vi "引用測試5.vi"() -> ()   [LabVIEW 2015]
uses:
  <vilib>/vision/Measure.llb/Edge Options.ctl
  <vilib>/vision/Measure.llb/Edge Polarity.ctl
  <vilib>/userdefined/High Color/IMAQdx.ctl
  <vilib>/vision/driver/NI_Vision_Acquisition_Software.lvlib
  <vilib>/vision/NI_Vision_Development_Module.lvlib
panel:
  out "Line Profile":T1(graph)
  out "Location (Pixel)":cluster{"X":sgl, "Y":sgl}
  in  "線":enum16{"Start to End", "End to Start"}(ring)
  in  "Session In":T2="cam0"
  out "output cluster":cluster{"Data name":string, "Data":variant}
  in  "Numeric":i32
  in  "ROI":T3=enum."Set Data"
  in  "動作":bool
  in  "重新開圖":bool
  out "Line Data":cluster{"X":sgl, "Y":sgl, "T":sgl}
  in  "開圖":bool
  in  "ShowData":bool
  in  "DieArea":i32=100 min=10
  in  "動作":enum16{"什麼也不做", "抓邊", "看灰階", "分析光源均勻度"}(ring)
  out "Mean":sgl format="%#.2f"
  out "Histogram":T4(graph)
  in  "取像":bool
  in  "Edge Options":T5={"Edge Polarity"=0, "Kernel Size"=3, "Width"=3, "Minimum Edge Strength"=10.0, "Interpolation Type"=enum."Bilinear Fixed", "Data Processing Method"=enum."Average"} {"Edge Polarity" items=["All Edges", "Rising Edges", "Falling Edges"]; "Minimum Edge Strength" format="%.2f"; "Width" step=2; "Kernel Size" step=2}
  out "error out":errorcluster
  out "Ellipse":T7 {"Minor Axis"."Point 2"."Y" format="%.2f"; "Minor Axis"."Point 2"."X" format="%.2f"; "Minor Axis"."Point 1"."Y" format="%.2f"; "Minor Axis"."Point 1"."X" format="%.2f"; "Major Axis"."Point 2"."Y" format="%.2f"; "Major Axis"."Point 2"."X" format="%.2f"; "Major Axis"."Point 1"."Y" format="%.2f"; "Major Axis"."Point 1"."X" format="%.2f"; "Center"."Y" format="%.2f"; "Center"."X" format="%.2f"}
  in  "圓":enum16{"Inner to Outer", "Outer to Inner"}(ring)
  out "Gradient Information":dbl[][](graph)
  in  "邊":T8(ring)
  in  "Process":T9(ring)
  in  "Gap":i32=10 min=1 max=300
  in  "stop":bool
  out "Image":T10(plugin-control)
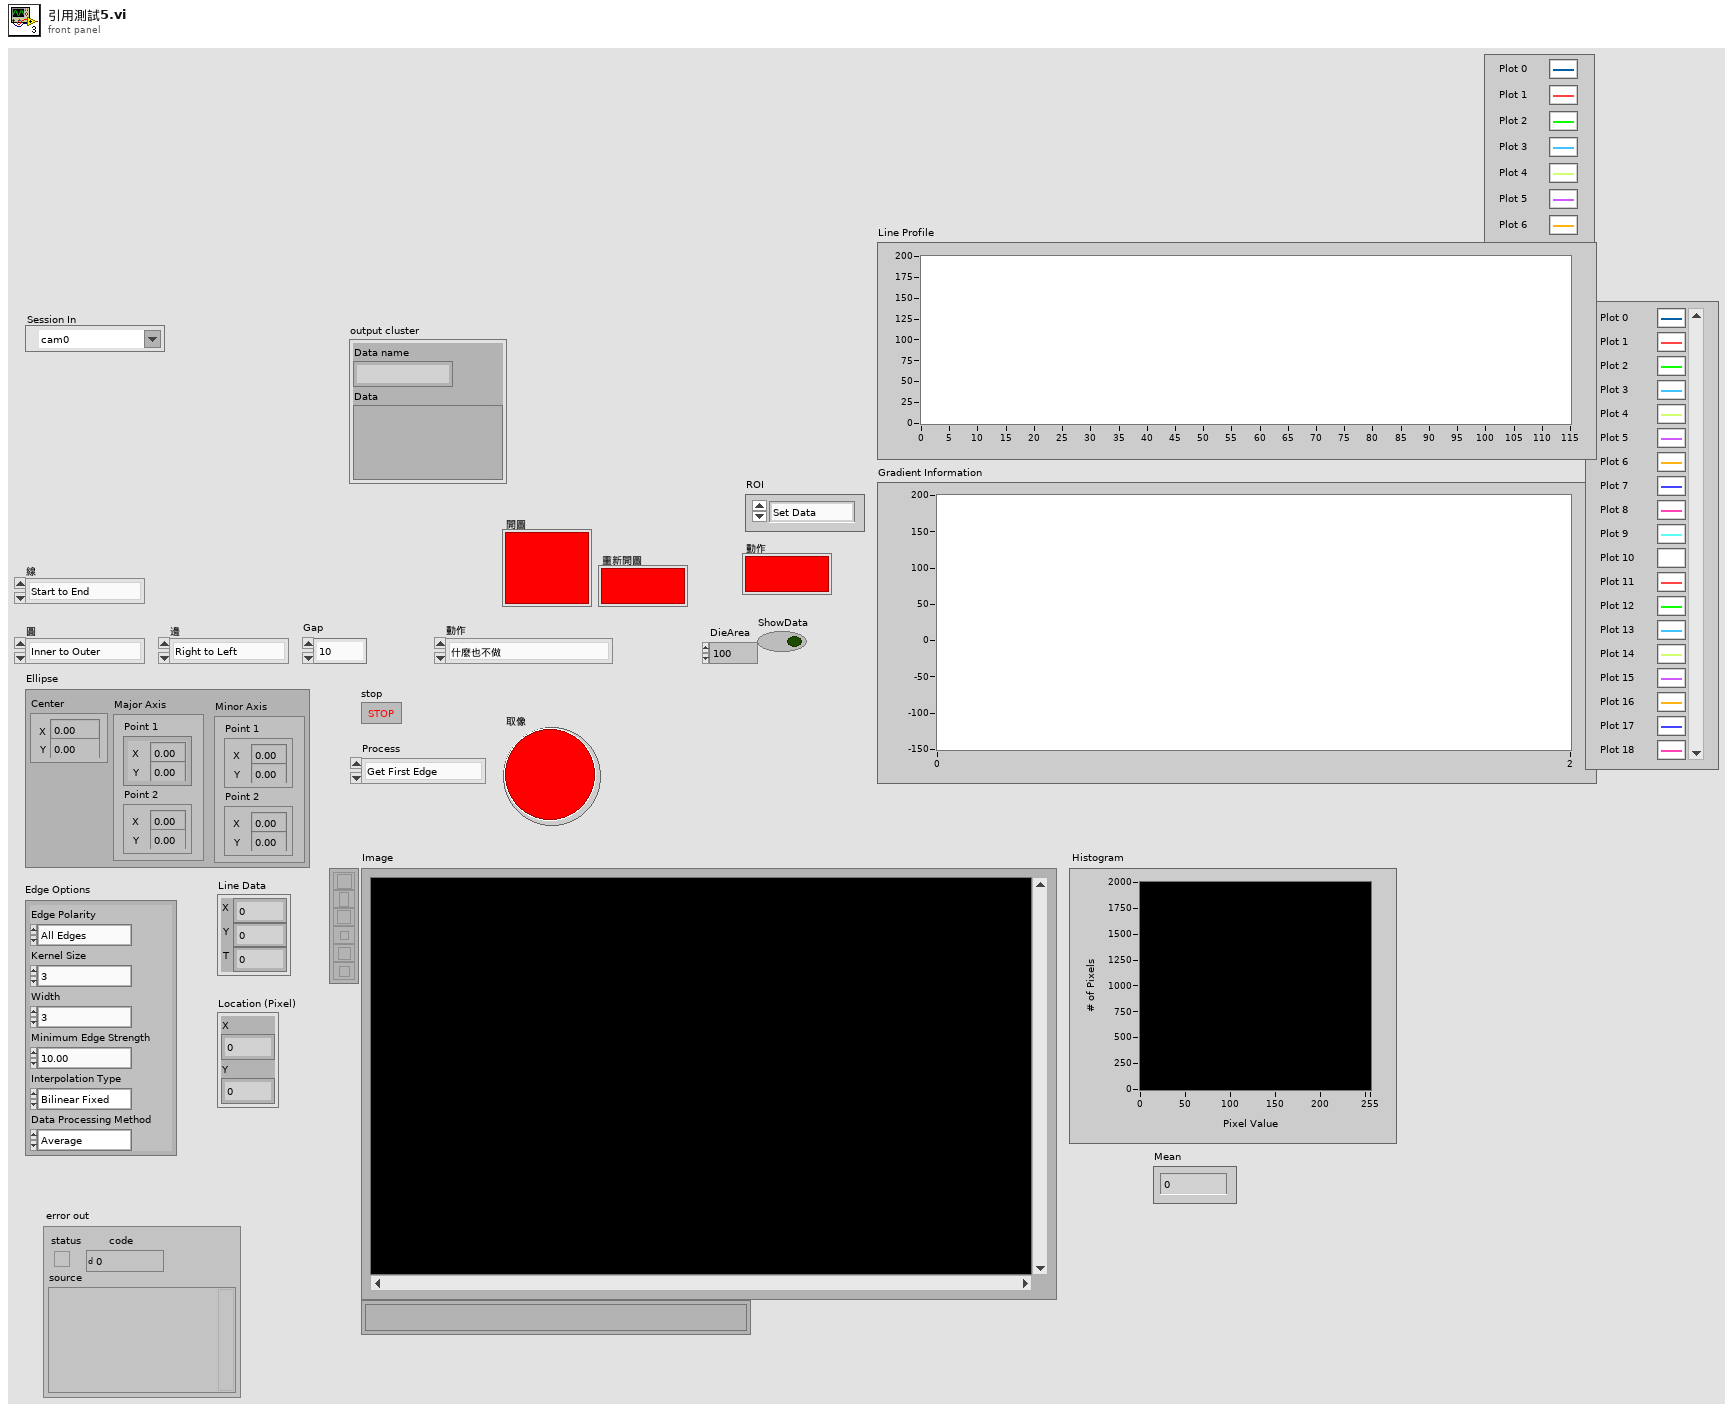
[diagram p1: front panel]
types:
  T1 = cluster{"x0":sgl, "dx":sgl, "Pixels Line":sgl[]}[]
  T2 = typedef "IMAQdx.ctl" = refnum<k21>
  T3 = typedef "Action_Data.ctl" = enum16{"Initialize", "Get Data", "Set Data", "Delete Data", "Idle"}
  T4 = cluster{"Starting Value":sgl, "Incremental Value":sgl, "Histogram":u32[]}
  T5 = typedef "Edge Options.ctl" = cluster{"Edge Polarity":T6, "Kernel Size":u32, "Width":u32, "Minimum Edge Strength":sgl, "Interpolation Type":enum32{"Zero Order", "Bilinear", "Quadratic", "Cubic", "Bilinear Fixed"}, "Data Processing Method":enum32{"Average", "Median"}}
  T6 = typedef "Edge Polarity.ctl" = u32
  T7 = cluster{"Center":cluster{"X":sgl, "Y":sgl}, "Major Axis":cluster{"Point 1":cluster{"X":sgl, "Y":sgl}, "Point 2":cluster{"X":sgl, "Y":sgl}}, "Minor Axis":cluster{"Point 1":cluster{"X":sgl, "Y":sgl}, "Point 2":cluster{"X":sgl, "Y":sgl}}}
  T8 = enum16{"Right to Left", "Left  to Right", "Up to Down", "Down to Up"}
  T9 = enum16{"Get First Edge", "Get First + Last Edge", "Get All Edges", "Get Best Edge"}
  T10 = typedef "IMAQ Image.ctl" = refnum<image>
  T11 = typedef "IMAQ Rectangle" = cluster{"Left":i32, "Top":i32, "Right":i32, "Bottom":i32, "Rotation":dbl}
  T12 = typedef "ROI Descriptor" = cluster{"Global Rectangle":i32[], "Contours":cluster{"ID":enum32{"External", "Internal"}, "Type":u32, "Coordinates":i32[]}[]}
  T13 = typedef "Image Type" = u32
  T14 = cluster{"Global Rectangle":i32[], "Contours":cluster{"Contour Type":u32, "ROI Type":u32, "Points":i32[]}[]}
  T15 = cluster{"Contour Type":u32, "ROI Type":u32, "Points":i32[]}[]
  T16 = cluster{"Contour Type":u32, "ROI Type":u32, "Points":i32[]}
  T17 = enum32{"Zero Order", "Bilinear", "Quadratic", "Cubic", "Bilinear Fixed"}
  T18 = cluster{"邊":enum16{"Right to Left", "Left  to Right", "Up to Down", "Down to Up"}, "動作":enum16{"什麼也不做", "抓邊", "看灰階", "分析光源均勻度"}, "圓":enum16{"Inner to Outer", "Outer to Inner"}, "Process":enum16{"Get First Edge", "Get First + Last Edge", "Get All Edges", "Get Best Edge"}, "ROI Type":u32, "Gap":i32, i32, i32, i32, i32, "Edge Polarity":T6, "Kernel Size":u32, "Width":u32, "Minimum Edge Strength":sgl, "Interpolation Type":enum32{"Zero Order", "Bilinear", "Quadratic", "Cubic", "Bilinear Fixed"}, "Data Processing Method":enum32{"Average", "Median"}, "DieArea":i32, "ShowData":bool, "線":enum16{"Start to End", "End to Start"}}
  T19 = cluster{"邊":bool, "動作":bool, "圓":bool, "Process":bool, "ROI Type":bool, "Gap":bool, bool, bool, bool, bool, "Edge Polarity":bool, "Kernel Size":bool, "Width":bool, "Minimum Edge Strength":bool, "Interpolation Type":bool, "Data Processing Method":bool, "DieArea":bool, "ShowData":bool, "線":bool}
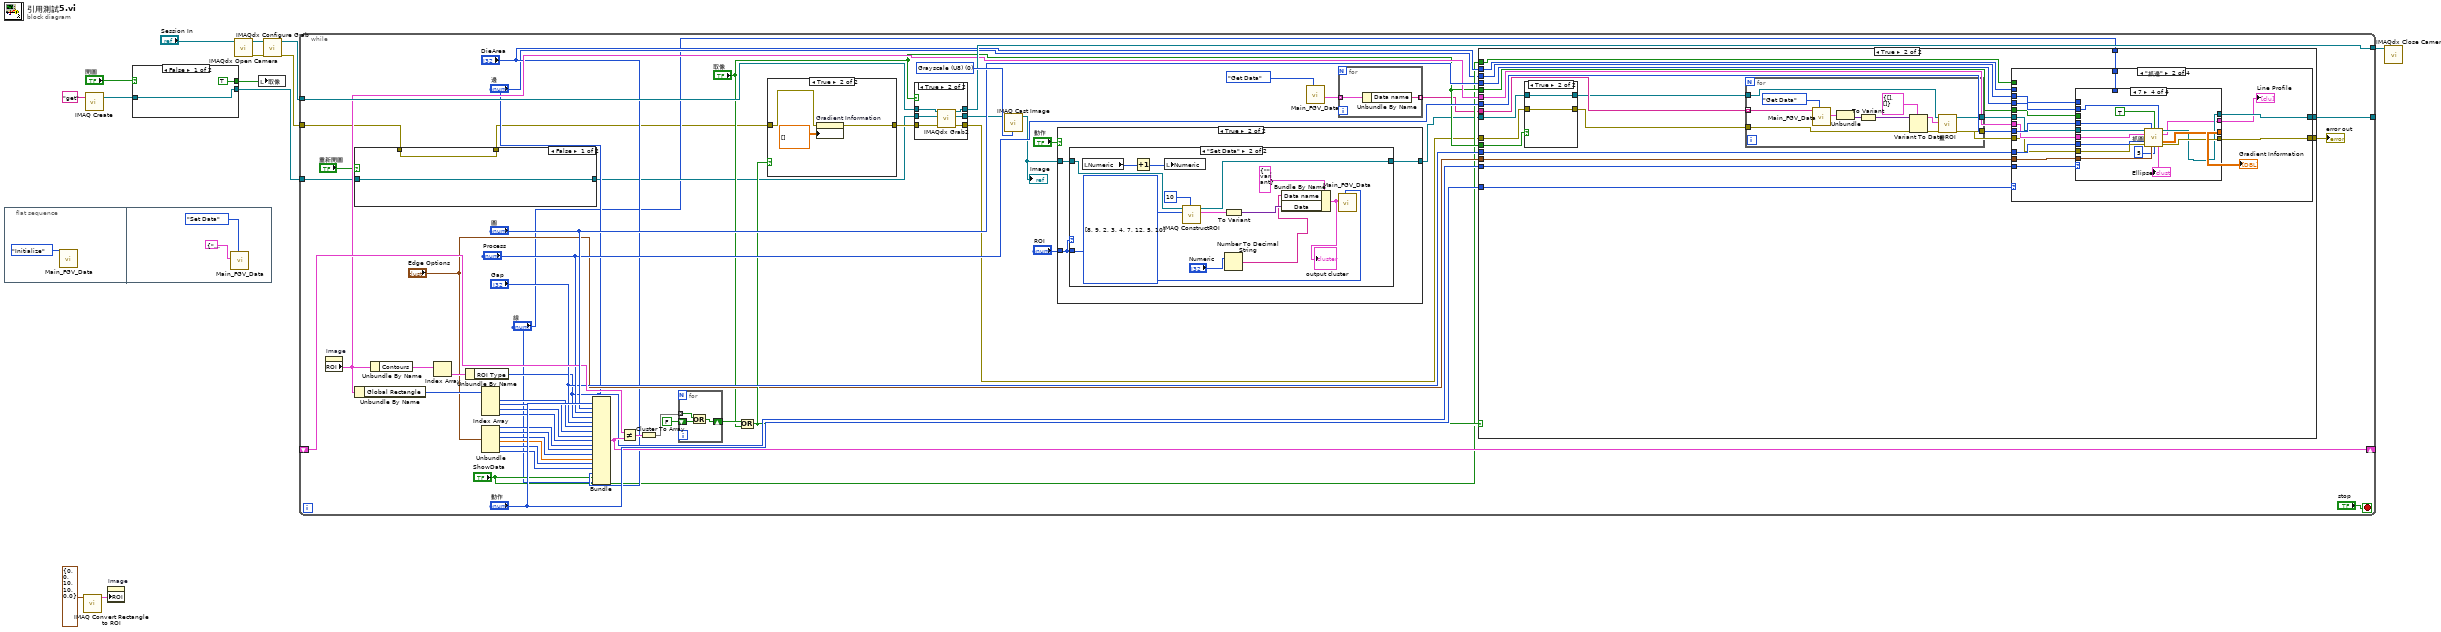
[diagram p0: block diagram]
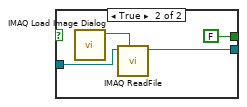
[diagram p2: hidden frame]
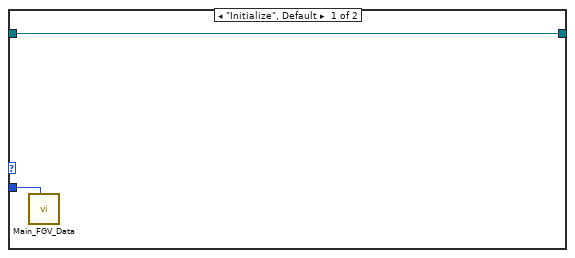
[diagram p4: hidden frame]
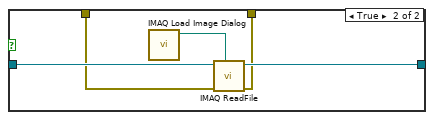
[diagram p5: hidden frame]
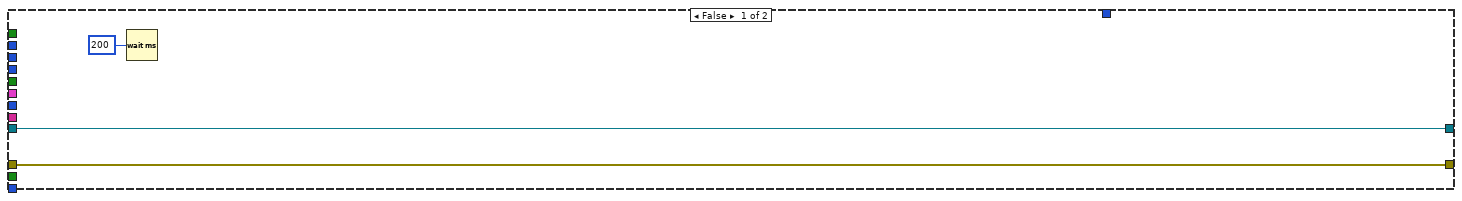
[diagram p7: hidden frame]
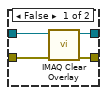
[diagram p8: hidden frame]
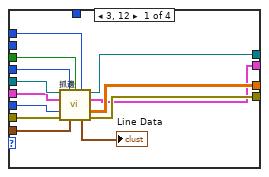
[diagram p10: hidden frame]
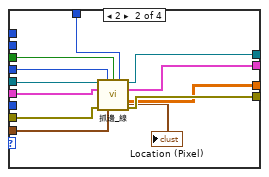
[diagram p11: hidden frame]
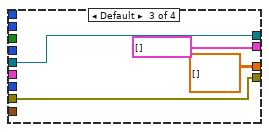
[diagram p12: hidden frame]
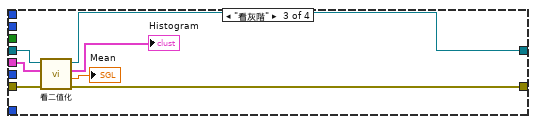
[diagram p13: hidden frame]
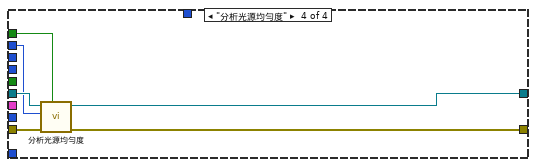
[diagram p14: hidden frame]
diagram:
  n1 = flat-sequence {
    frame #0 {
      n2 = call "Main_FGV_Data.vi"("Action_Data"=Action_Data."Initialize") -> ()  [unwired: 9 in, 2 out]
    }
    frame #1 {
      n3 = call "Main_FGV_Data.vi"("Action_Data"=Action_Data."Set Data", "Data In"=cluster{"Data name":string, "Data":variant} {"Data name"="Oringal", "Data"=variant(cluster{"Global Rectangle":i32[], "Contours":cluster{"ID":enum32{"External", "Internal"}, "Type":u32, "Coordinates":i32[]}[]} {"Global Rectangle"=[0, 959, 2, 960], "Contours"=[{"ID"=enum."External", "Type"=2, "Coordinates"=[0, 959, 1, 959]}]})} ("output cluster 3")) -> ()  [unwired: 8 in, 2 out]
    }
  }
  n4 = call "IMAQ Convert Rectangle to ROI"("Rectangle"=T11 {"Left"=0, "Top"=0, "Right"=10, "Bottom"=10, "Rotation"=0.0}) -> ("ROI Descriptor"=w6:T12)  [unwired: 8 in, 1 out]
  n5 = call "IMAQ Create"("Image Name"="get") -> ("New Image"=w3:T10)  [unwired: 4 in, 1 out]
  n6 = property on="Image" class="ImageControl"("ROI"=w6) -> ()  [unwired: 2 in, 2 out]
  n7 = case shown="False" "開圖" {
    tunnel: [TRUE ("取像") FALSE ("取像")] -> w4
    tunnel: w3 -> [w17 w21]
    tunnel: [w17 w20] -> w2
    frame False {
    }
    frame True {
      n8 = call "IMAQ Load Image Dialog"() -> ("Path"=w19:path)  [unwired: 9 in, 2 out]
      n9 = call "IMAQ ReadFile"("File Path"=w19, "Image"=w21) -> ("Image Out"=w20:T10)  [unwired: 5 in, 4 out]
    }
  }
  n10 = call <vilib>:"IMAQdx Open Camera.vi"("Session In"="Session In") -> ("error out"=w8:errorcluster, "Session Out"=w9:T2)  [unwired: 9 in]
  n11 = local write "取像"(w4) -> ()
  n12 = call <vilib>:"IMAQdx Configure Grab.vi"("error in"=w8, "Session In"=w9) -> ("error out"=w1:errorcluster, "Session Out"=w12:T2)  [unwired: 8 in]
  n13 = while {
    tunnel: w12 -> [w75]
    tunnel: w2 -> [w35]
    tunnel: [w57] -> w11
    tunnel: [w71] -> _
    shift-right: [w66] -> _
    shift-left: _ -> [w65]
    tunnel: w1 -> [w24]
    stop <- "stop" stop-if-true
    w73 = T13 0 items=["Grayscale (U8)", "Grayscale (I16)", "Grayscale (SGL)", "Complex (CSG)", "RGB (U32)", "HSL (U32)", "RGB (U64)", "Grayscale (U16)"] ("Image Type")
    n14 = property on="Image" class="ImageControl"() -> ("ROI"=w55:T14)  [unwired: 2 in, 2 out]
    n15 = case shown="False" "重新開圖" {
      tunnel: w35 -> [w98 w101]
      tunnel: [w98 w102] -> w34
      tunnel: w24 -> [w97 w100]
      tunnel: [w97 w99] -> w23
      frame False {
      }
      frame True {
        n16 = call "IMAQ Load Image Dialog"() -> ("Path"=w103:path)  [unwired: 9 in, 2 out]
        n17 = call "IMAQ ReadFile"("File Path"=w103, "error in (no error)"=w100, "Image"=w101) -> ("error out"=w99:errorcluster, "Image Out"=w102:T10)  [unwired: 4 in, 3 out]
      }
    }
    n18 = Unbundle By Name(w55) -> ("Global Rectangle"=w54:i32[])
    n19 = Unbundle By Name(w55) -> ("Contours"=w70:T15)
    n20 = Index Array(array=w70) -> (element=w69:T16)  [unwired: 1 in]
    n21 = Unbundle By Name(w69) -> ("ROI Type"=w59:u32)
    n22 = Index Array(array=w54) -> (element #1=w53:i32, element #2=w52:i32, element #3=w51:i32, element #4=w50:i32)  [unwired: 4 in]
    n23 = Unbundle("Edge Options") -> ("Edge Polarity"=w47:T6, "Kernel Size"=w46:u32, "Width"=w45:u32, "Minimum Edge Strength"=w44:sgl, "Interpolation Type"=w43:T17, "Data Processing Method"=w42:enum32{"Average", "Median"})
    n24 = Bundle("邊"="邊", "動作"="動作", "圓"="圓", "Process"="Process", "ROI Type"=w59, "Gap"="Gap", w53, w52, w51, w50, "Edge Polarity"=w47, "Kernel Size"=w46, "Width"=w45, "Minimum Edge Strength"=w44, "Interpolation Type"=w43, "Data Processing Method"=w42, "DieArea"="DieArea", "ShowData"="ShowData", "線"="線") -> (w66:T18)  [unwired: 1 in]
    n25 = Not Equal?(x=w65, y=w66) -> (x != y?=w58:T19)
    n26 = Cluster To Array(cluster=w58) -> (array=w64:bool[])
    n27 = for {
      tunnel: w64 -> [w110] mode=indexing
      shift-right: [w109] -> w62
      shift-left: FALSE -> [w108]
      n28 = Or(x=w110, y=w108) -> (x .or. y?=w109:bool)
    }
    n29 = Or(x=w62, y="取像") -> (x .or. y?=w49:bool)
    n30 = case shown="True" w49 {
      tunnel: [w104 w106] -> w72
      tunnel: w23 -> [w104 w105]
      frame False {
      }
      frame True {
        n31 = property on="Gradient Information" class="WFChart (strict)"(error in=w105, "History Data"=dbl[][] []) -> (error out=w106:errorcluster)  [unwired: 1 in, 1 out]
      }
    }
    n32 = case shown="True" "取像" {
      tunnel: w75 -> [w229 w235]
      tunnel: w34 -> [w228 w234]
      tunnel: [w229 w233] -> w57
      tunnel: [w228 w232] -> w56
      tunnel: w72 -> [w227 w231]
      tunnel: [w227 w230] -> w28
      frame False {
      }
      frame True {
        n33 = call <vilib>:"IMAQdx Grab2.vi"("error in"=w231, "Image In"=w234, "Session In"=w235) -> ("error out"=w230:errorcluster, "Image Out"=w232:T10, "Session Out"=w233:T2)  [unwired: 5 in, 1 out]
      }
    }
    n34 = call "IMAQ Cast Image"("Image Type"=w73, "Image Src"=w56) -> ("Image Dst Out"=w27:T10)  [unwired: 8 in, 1 out]
    "Image" <- w27
    n35 = case shown="True" "動作" {
      tunnel: w27 -> [w78 w81]
      tunnel: [w78 w80] -> w26
      tunnel: "ROI" -> [_ w79]
      frame False {
      }
      frame True {
        n36 = case shown="\"Set Data\"" w79 {
          tunnel: w81 -> [w83 w94]
          tunnel: [w83 w92] -> w80
          tunnel: w79 -> [w82 w86]
          frame "Initialize", Default {
            n37 = call "Main_FGV_Data.vi"("Action_Data"=w82) -> ()  [unwired: 9 in, 2 out]
          }
          frame "Set Data" {
            w96 = u32[] [8, 9, 2, 3, 4, 7, 12, 5, 10] items=["No Selection", "Point", "Line", "Rectangle", "Oval", "Polygon", "Freehand Region", "Annulus", "Zoom", "Pan", "Broken Line", "Freehand Line", "Rotated Rectangle"] ("Tools")
            n38 = local read "Numeric"() -> (w88:i32)
            n39 = Increment(x=w88) -> (x+1=w87:i32)
            n40 = local write "Numeric"(w87) -> ()
            n41 = call "IMAQ ConstructROI"("Window Number (-1...15)"=10, "Tools"=w96, "Image"=w94) -> ("ROI Descriptor Out"=w93:T12, "Image Out (duplicate)"=w92:T10)  [unwired: 5 in, 2 out]
            n42 = To Variant(anything=w93) -> (Variant=w91:variant)
            n43 = Number To Decimal String(number="Numeric") -> (decimal integer string=w85:string)  [unwired: 1 in]
            n44 = Bundle By Name(cluster=cluster{"Data name":string, "Data":variant} {"Data name"="", "Data"=variant} ("Data In"), "Data name"=w85, "Data"=w91) -> (w84:cluster{"Data name":string, "Data":variant})
            "output cluster" <- w84
            n45 = call "Main_FGV_Data.vi"("Action_Data"=w86, "Data In"=w84) -> ()  [unwired: 8 in, 2 out]
          }
        }
      }
    }
    n46 = call "Main_FGV_Data.vi"("Action_Data"=Action_Data."Get Data") -> ("Data Array out"=w32:cluster{"Data name":string, "Data":variant}[])  [unwired: 9 in, 1 out]
    n47 = for {
      tunnel: [w77] -> w29 mode=indexing
      tunnel: w32 -> [w76] mode=indexing
      n48 = Unbundle By Name(w76) -> ("Data name"=w77:string)
    }
    n49 = case shown="True" w49 {
      tunnel: "Gap" -> [_ w135]
      tunnel: w28 -> [w113 w120]
      tunnel: "Process" -> [_ w134]
      tunnel: w26 -> [w112 w125]
      tunnel: [w112 w133] -> w71
      tunnel: w55 -> [_ w132]
      tunnel: w59 -> [_ w131]
      tunnel: "Edge Options" -> [_ w130]
      tunnel: [w113 w129] -> w38
      tunnel: "動作" -> [_ w128]
      tunnel: "圓" -> [_ w127]
      tunnel: "取像" -> [_ w126]
      tunnel: "取像" -> [_ w124]
      tunnel: "DieArea" -> [_ w123]
      tunnel: "ShowData" -> [_ w122]
      tunnel: "邊" -> [_ w121]
      tunnel: w29 -> [_ w118]
      tunnel: "線" -> [_ w114]
      frame False {
        n50 = Wait (ms)(milliseconds to wait=u32 200) -> ()  [unwired: 1 out]
      }
      frame True {
        n51 = case shown="True" w126 {
          tunnel: w125 -> [w150 w153]
          tunnel: [w151 w153] -> w116
          tunnel: w120 -> [w149 w152]
          tunnel: [w148 w152] -> w117
          frame False {
            n52 = call "IMAQ Clear Overlay"("error in (no error)"=w149, "Image"=w150) -> ("error out"=w148:errorcluster, "Image Out"=w151:T10)  [unwired: 8 in]
          }
          frame True {
          }
        }
        n53 = for {
          tunnel: w116 -> [w147]
          tunnel: [w146] -> w115
          tunnel: w117 -> [w137]
          tunnel: [w136] -> w119
          tunnel: w118 -> [w138] mode=indexing
          n54 = call "Main_FGV_Data.vi"("Action_Data"=Action_Data."Get Data", "Data name"=w138) -> ("Data  Out"=w144:cluster{"Data name":string, "Data":variant})  [unwired: 8 in, 1 out]
          n55 = Unbundle(w144) -> ("Data"=w143:variant)  [unwired: 1 out]
          n56 = To Variant(anything=w143) -> (Variant=w142:variant)
          n57 = Variant To Data(error in=w137, type=T12 {"Global Rectangle"=[], "Contours"=[]} ("ROI Descriptor"), Variant=w142) -> (data=w140:T12, error out=w139:errorcluster)
          n58 = call "畫ROI.vi"("error in (no error)"=w139, "ROI In"=w140, "Image In"=w147) -> ("error out"=w136:errorcluster, "Image Out"=w146:T10)  [unwired: 7 in]
        }
        n59 = case shown="\"抓邊\"" w128 {
          tunnel: w135 -> [_ w170 _ _]
          tunnel: w119 -> [w154 w158 w217 w222]
          tunnel: w127 -> [_ w169 _ _]
          tunnel: w134 -> [_ w168 _ _]
          tunnel: w115 -> [w155 w167 w219 w224]
          tunnel: [w155 w166 w220 w225] -> w133
          tunnel: w132 -> [_ w165 w218 _]
          tunnel: w131 -> [_ w164 _ _]
          tunnel: w130 -> [_ w163 _ _]
          tunnel: [w154 w161 w214 w226] -> w129
          tunnel: w124 -> [_ w160 _ _]
          tunnel: w123 -> [_ _ _ w223]
          tunnel: w122 -> [_ _ _ w221]
          tunnel: w121 -> [_ w159 _ _]
          tunnel: w114 -> [_ w157 _ _]
          frame "什麼也不做", Default {
          }
          frame "抓邊" {
            n60 = case shown="7" w164 {
              tunnel: w165 -> [w182 w195 _ w209]
              tunnel: w170 -> [w181 _ _ w210]
              tunnel: w158 -> [w180 w193 w197 w211]
              tunnel: w169 -> [_ _ _ w206]
              tunnel: w168 -> [w175 w190 _ w207]
              tunnel: [w178 w187 dbl[][] [] ("Gradient Information") w213] -> w162
              tunnel: w167 -> [w183 w194 w199 w208]
              tunnel: [w177 w191 w199 w202] -> w166
              tunnel: [w179 w192 w197 w204] -> w161
              tunnel: w163 -> [w176 w186 _ w212]
              tunnel: w160 -> [w174 w189 _ _]
              tunnel: w159 -> [w172 _ _ _]
              tunnel: w157 -> [_ w188 _ _]
              tunnel: [w171 w184 T1 [] ("Line Profile") w200] -> w156
              frame 3, 12 {
                n61 = call "抓邊.vi"("Image In"=w183, "Process"=w175, "Optimized Mode"=w174, "Direction"=w172, "ROI"=w182, "Gap"=w181, "error In"=w180, "Edge Options"=w176) -> ("Image Out"=w177:T10, "Line Profile"=w171:T1, "Gradient Information"=w178:dbl[][], "Line Data"=→"Line Data":cluster{"X":sgl, "Y":sgl, "T":sgl}, "error out"=w179:errorcluster)  [unwired: 3 in]
              }
              frame 2 {
                n62 = call "抓邊_線.vi"("Image In"=w194, "Process"=w190, "Optimized Mode"=w189, "Direction"=w188, "ROI"=w195, "error In"=w193, "Edge Options"=w186) -> ("Image Out"=w191:T10, "Line Profile"=w184:T1, "Gradient Information"=w187:dbl[][], "Location (Pixel)"=→"Location (Pixel)":cluster{"X":sgl, "Y":sgl}, "error out"=w192:errorcluster)  [unwired: 4 in]
              }
              frame Default {
              }
              frame 7 {
                n63 = call "抓圓.vi"("Image In"=w208, "Process"=w207, "Optimized Mode"=TRUE, "Direction"=w206, "ROI"=w209, "Gap"=w210, "error In"=w211, "Edge Options"=w212, "Point Diameter (5)"=u32 5) -> ("Imag e Out"=w202:T10, "Line Profile"=w200:T1, "Gradient Information"=w213:dbl[][], "Ellipse"=→"Ellipse":T7, "error out"=w204:errorcluster)  [unwired: 2 in]
              }
            }
            "Gradient Information" <- w162
            "Line Profile" <- w156
          }
          frame "看灰階" {
            n64 = call "看二值化.vi"("error in (no error)"=w217, "ROI Descriptor"=w218, "Image In"=w219) -> ("error out"=w214:errorcluster, "Mean"=→"Mean":sgl, "Histogram"=→"Histogram":T4, "Image Out"=w220:T10)  [unwired: 4 in, 1 out]
          }
          frame "分析光源均勻度" {
            n65 = call "分析光源均勻度.vi"("ShowData"=w221, "error in (no error)"=w222, "DieArea"=w223, "Image In"=w224) -> ("error out"=w226:errorcluster, "Image"=w225:T10)  [unwired: 6 in]
          }
        }
      }
    }
    "error out" <- w38
  }
  n66 = call <vilib>:"IMAQdx Close Camera.vi"("Session In"=w11) -> ()  [unwired: 10 in, 1 out]
